vi "Test.vi"() -> ()   [LabVIEW 2021, in "Test.lvlib"]
uses:
  <resource>/plugins/NIIconEditor/UI/Harness/Test.lvlib
  <resource>/plugins/IconEditorInterface.lvlibp/_IconEditorInterface.lvclass
panel:
  in  "class path":path=path "C:/git/labview-icon-editor/resource/plugins/NIIconEditor/UI/Default/IconEditorDefaultPlugin.lvclass"
  out "error out":errorcluster
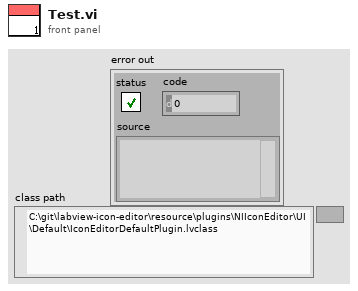
[diagram p1: front panel]
types:
  T1 = cluster{"image type":i32, "image depth":i32, "image":u8[], "mask":u8[], "colors":u32[], "Rectangle":cluster{"left":i16, "top":i16, "right":i16, "bottom":i16}}
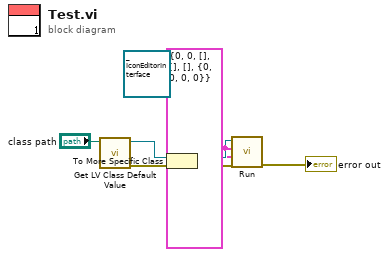
[diagram p0: block diagram]
diagram:
  w2 = T1 {"image type"=0, "image depth"=0, "image"=[], "mask"=[], "colors"=[], "Rectangle"={"left"=0, "top"=0, "right"=0, "bottom"=0}} ("Color icon in")
  n1 = call <vilib>:"Get LV Class Default Value.vi"("class path"="class path") -> ("error out"=w7:errorcluster, "object"=w6:refnum<class>)  [unwired: 9 in]
  n2 = To More Specific Class(target class=refnum<class "_IconEditorInterface.lvclass"> refnum ("IconEditorInterface.lvlibp:_IconEditorInterface.lvclass"), reference=w6, error in=w7) -> (specific class reference=w3:refnum<class "_IconEditorInterface.lvclass">, error out=w4:errorcluster)
  n3 = call-dynamic "Run.vi"("error in (no error)"=w4, "BW icon in"=w2, "Color icon in"=w2, "IconEditorInterface in"=w3) -> ("error out"=→"error out":errorcluster)  [unwired: 3 in, 4 out]
